vi "Bulk Add AI Register Dialog.vi"(8 "error in (no error)":errorcluster) -> (0 "error out":errorcluster, 1 "Cancelled?":bool, 2 "Quantity Out":u16, 3 "Root Name Out":string, 4 "DataType Out":T1, 5 "Starting Address Out":u16, 7 "Pack Values? Out":bool)   [LabVIEW 2015, in "Modbus Master System Explorer.lvlib"]
uses:
  Modbus Master System Explorer.lvlib
  Shared/Controls/Data Model/DataType.ctl
  Shared/Modbus Master Shared.lvlib
panel:
  in  "Pack Values?":bool
  in  "DataType":T1=enum."U16"
  in  "Cancel Button":bool
  in  "OK Button":bool
  in  "Quantity":u16
  in  "Starting Address":u16
  in  "Root Name":string="Input Register"
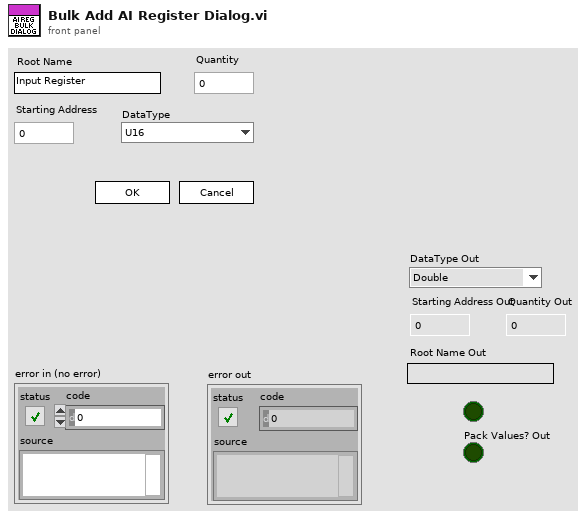
[diagram p1: front panel]
types:
  T1 = typedef "Modbus Master Shared.lvlib/DataType.ctl" = enum16{"Double", "Single", "I64", "I32", "I16", "I8", "U64", "U32", "U16", "U8", "Boolean"}
  T2 = enum32{"Invalid", "Standard", "Closed", "Hidden", "Minimized", "Maximized"}
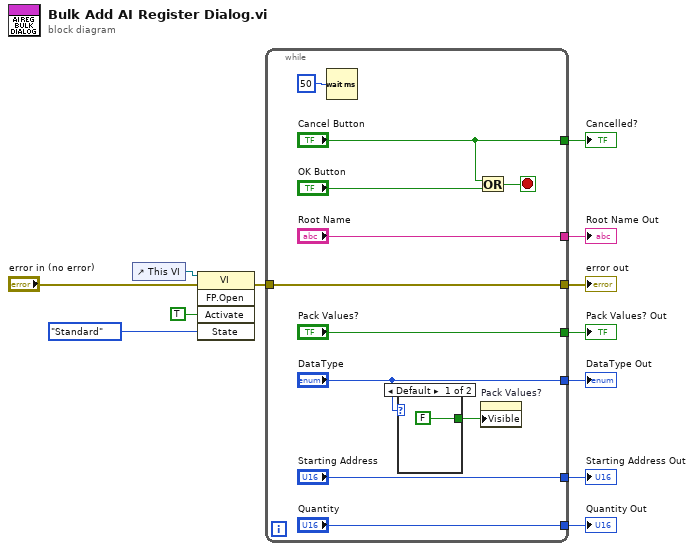
[diagram p0: block diagram]
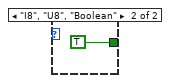
[diagram p2: hidden frame]
diagram:
  n1 = control-ref of="This VI"() -> (w8:refnum<vi>)
  n2 = invoke class="VI" method="FP.Open"(reference=w8, error in="error in (no error)", "Activate"=TRUE ("Activate?"), "State"=T2."Standard") -> (error out=w4:errorcluster)  [unwired: 1 in, 4 out]
  n3 = while {
    tunnel: ["Cancel Button"] -> w12
    tunnel: ["Root Name"] -> w11
    tunnel: ["Quantity"] -> w10
    tunnel: ["Starting Address"] -> w9
    tunnel: w4 -> [w16]
    tunnel: [w16] -> w3
    tunnel: ["DataType"] -> w2
    tunnel: ["Pack Values?"] -> w1
    stop <- w22 stop-if-true
    n4 = Wait (ms)(milliseconds to wait=u32 50) -> ()  [unwired: 1 out]
    n5 = case shown="Default" "DataType" {
      tunnel: [FALSE ("Visible") TRUE ("Visible")] -> w13
      frame Default {
      }
      frame "I8", "U8", "Boolean" {
      }
    }
    n6 = Or(x="Cancel Button", y="OK Button") -> (x .or. y?=w22:bool)
    n7 = property on="Pack Values?" class="Bool (strict)"("Visible"=w13) -> ()  [unwired: 2 in, 2 out]
  }
  "error out" <- w3
  "Root Name Out" <- w11
  "Starting Address Out" <- w9
  "Cancelled?" <- w12
  "Quantity Out" <- w10
  "DataType Out" <- w2
  "Pack Values? Out" <- w1
